vi "ProData.vi"() -> (3 "ProDataQueue":T1)   [LabVIEW 2018]
uses:
  ProDataQueue.ctl
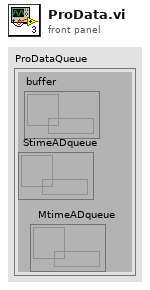
[diagram p1: front panel]
types:
  T1 = typedef "ProDataQueue.ctl" = cluster{"buffer ":refnum<queue>, " StimeADqueue":refnum<queue>, "  MtimeADqueue":refnum<queue>}
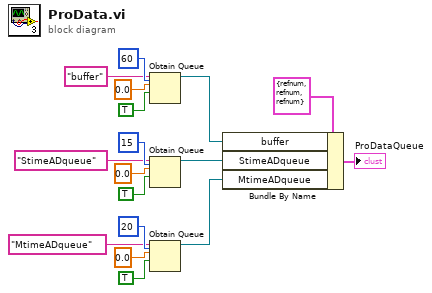
[diagram p0: block diagram]
diagram:
  n1 = Obtain Queue(max queue size (-1, unlimited)=60 ("队列最大值（-1，无限）"), name (unnamed)="buffer" ("名称（未命名）"), element data type=0.0, create if not found? (T)=TRUE ("如未找到则创建？(T)")) -> (queue out=w14:refnum<queue>)  [unwired: 1 in, 2 out]
  n2 = Obtain Queue(max queue size (-1, unlimited)=15 ("队列最大值（-1，无限）"), name (unnamed)="StimeADqueue" ("名称（未命名）"), element data type=0.0, create if not found? (T)=TRUE ("如未找到则创建？(T)")) -> (queue out=w15:refnum<queue>)  [unwired: 1 in, 2 out]
  n3 = Obtain Queue(max queue size (-1, unlimited)=20 ("队列最大值（-1，无限）"), name (unnamed)="MtimeADqueue" ("名称（未命名）"), element data type=0.0, create if not found? (T)=TRUE ("如未找到则创建？(T)")) -> (queue out=w17:refnum<queue>)  [unwired: 1 in, 2 out]
  n4 = Bundle By Name(cluster=T1 {"buffer "=refnum, " StimeADqueue"=refnum, "  MtimeADqueue"=refnum}, "buffer"=w14, "StimeADqueue"=w15, "MtimeADqueue"=w17) -> (→"ProDataQueue":T1)
